vi "Read.vi"(11 "Log Status Value in":refnum<class "Log Status Value.lvclass">) -> (2 "Log Status":T1)   [LabVIEW 2020, in "VolatusData.lvlib" / "Log Status Value.lvclass"]
uses:
  Log Status Value.lvclass
  Log Status Value.lvclass/Log Status Value.ctl
  Logging State.ctl
  VolatusData.lvlib
  Log Status.ctl
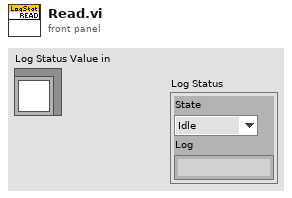
[diagram p1: front panel]
types:
  T1 = typedef "VolatusData.lvlib/Log Status.ctl" = cluster{"State":T2, "Log":string}
  T2 = typedef "VolatusData.lvlib/Logging State.ctl" = enum16{"Idle", "Starting", "Logging", "Stopping"}
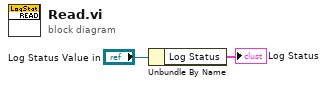
[diagram p0: block diagram]
diagram:
  n1 = Unbundle By Name("Log Status Value in") -> ("Log Status"=→"Log Status":T1)
